vi "SLM Ctrl Update Mode Names.vi"(7 "ModeNamesArray":T1, 13 "Number of Modes":i32) -> (8 "Mode Names":string[](array[string]))   [LabVIEW 2018]
uses:
  SLM Control TypeDefs/SLM Ctrl Mode Names.ctl
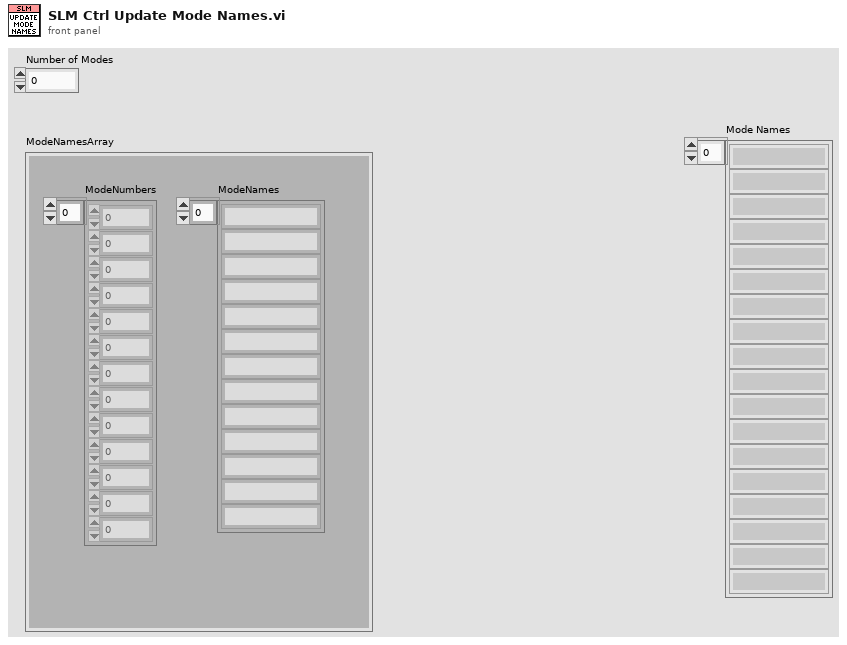
[diagram p1: front panel]
types:
  T1 = typedef "SLM Ctrl Mode Names.ctl" = cluster{"ModeNumbers":i32[], "ModeNames":string[]}
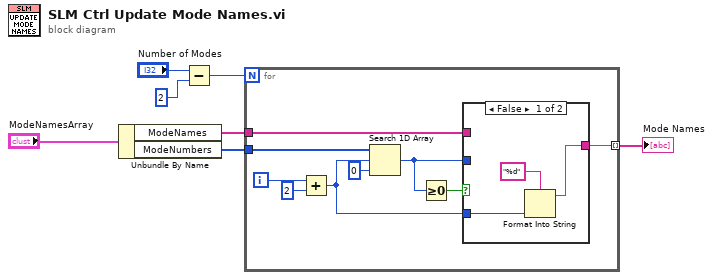
[diagram p0: block diagram]
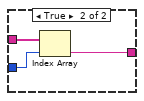
[diagram p2: hidden frame]
diagram:
  n1 = Unbundle By Name("ModeNamesArray") -> ("ModeNames"=w5:string[], "ModeNumbers"=w6:i32[])
  n2 = Subtract(x="Number of Modes", y=2) -> (x-y=w1:i32)
  n3 = for {
    N: w1 -> [_]
    tunnel: w6 -> [w16]
    tunnel: w5 -> [w14]
    tunnel: [w11] -> w4 mode=indexing
    i -> [w8]
    n4 = Add(x=w8, y=2) -> (x+y=w9:i32)
    n5 = Search 1D Array(1D array=w16, element=w9, start index (0)=0) -> (index of element=w12:i32)
    n6 = Greater Or Equal To 0?(x=w12) -> (x >= 0?=w13:bool)
    n7 = case shown="False" w13 {
      tunnel: w14 -> [_ w22]
      tunnel: w12 -> [_ w21]
      tunnel: [w17 w20] -> w11
      tunnel: w9 -> [w19 _]
      frame False {
        n8 = Format Into String(format string="%d", w19) -> (resulting string=w17:string)  [unwired: 2 in, 1 out]
      }
      frame True {
        n9 = Index Array(array=w22, index=w21) -> (element=w20:string)
      }
    }
  }
  "Mode Names" <- w4
